vi "Get Cold Block Temperature.vi"(8 "error in (no error)":errorcluster, 11 "Syringe Line in":refnum<class "Syringe Line.lvclass">) -> (0 "error out":errorcluster, 1 "Temperature (C)":dbl, 3 "Syringe Line out":refnum<class "Syringe Line.lvclass">, 4 "Frozen?":bool)   [LabVIEW 2015, in "cRIO-Carbondioxide.lvlib" / "CO2-Actor.lvlib" / "Syringe Line.lvclass"]
uses:
  Syringe Line.lvclass
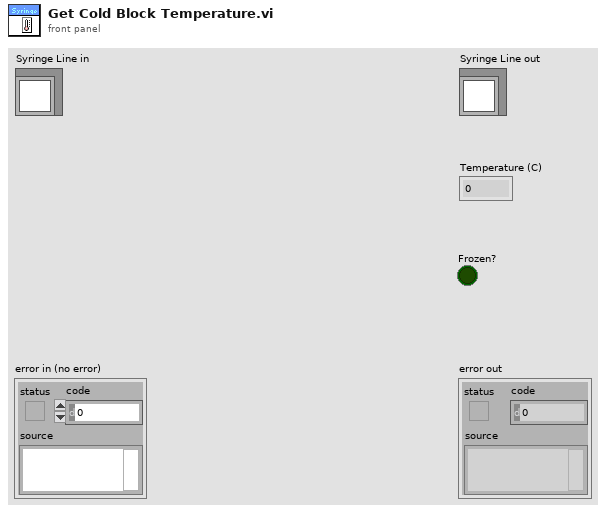
[diagram p1: front panel]
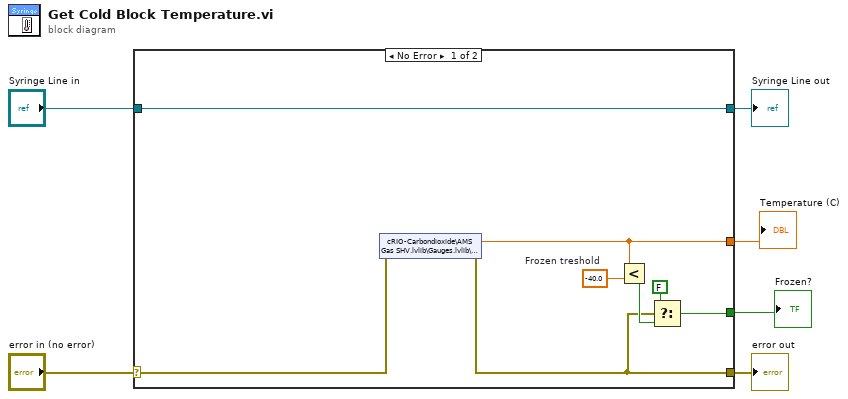
[diagram p0: block diagram]
diagram:
  n1 = case shown="No Error" "error in (no error)" {
    selector: "error in (no error)" -> [w13 w16]
    tunnel: [w9 w16] -> w5
    tunnel: [w14 w15] -> w3
    tunnel: "Syringe Line in" -> [w14 w15]
    tunnel: [w8 _] -> w2
    tunnel: [w7 _] -> w1
    frame No Error {
      w10 = -40.0  # Frozen treshold
      n2 = shared-variable "cRIO-Carbondioxide\\AMS Gas SHV.lvlib\\Gauges.lvlib\\Syringe TC"(error in=w13) -> (w7:dbl, error out=w9:errorcluster)
      n3 = Less?(x=w7, y=w10) -> (x < y?=w11:bool)
      n4 = Select(t=FALSE, s=w9, f=w11) -> (s? t:f=w8:bool)
    }
    frame Error {
    }
  }
  "error out" <- w5
  "Syringe Line out" <- w3
  "Frozen?" <- w2
  "Temperature (C)" <- w1
